vi "NNPC_Eval.vi"(4 "Eval Config":T1={"Extract Good Pixels from Bad"=FALSE, "# bins"=100}, 6 "Dataset(In3D_Out3D)":T28, 8 "error in":errorcluster, 9 "anomaly maps":sgl[][][](array[numeric]), 10 "pred scores":sgl[](array[numeric]), 11 "PCore_Instance in":T2={"Dataset_Stats"={"means"={"R"=0.0, "G"=0.0, "B"=0.0}, "vars"={"R"=0.0, "G"=0.0, "B"=0.0}, "DS_Size"=0}, "NN"={"Name"="", "No of Layers"=0, "mBatch"=0, "Layers"=[], "Dimty"=enum."In1D_Out1D", "Dims_In"={"C"=0, "H"=0, "W"=0}, "Dims_Out"={"C"=0, "H"=0, "W"=0}, "Working_Dir"=path "", "Train?"=FALSE, "Train_Params"={"Optimizer"=enum."SGD", "Beta_1"=0.0, "Beta_2"=0.0, "Weight Decay(L1)"=0.0, "Weight Decay(L2)"=0.0, "Data_Sampling"=enum."Random"}, "LR_Update_Policy"={"Policy_Type"=enum."Manual", "LR0"=0.0, "k"=0.0, "WarmUp_Policy"=enum."Step", "WarmUp_Iter"=0, "WarmUp_Ratio"=0.0}, "Session Data"={"Epochs"=0.0, "Tot_Iter"=0, "LR"=0.0, "LR_iter"=0}, "Ground_truth"={"Y"=variant}, "NNg_hdls"={"cudnn"=0, "cublas"=0, "stream"=0, "curand"=0}, "NN_Device"=enum."CPU", "GPU Id"=0, "Labels"=[], "Receptive Field"=[], "Loss_Type"=enum."None", "Loss_Cfg_Prms"=variant, "NNG_WS"={"NNG_WS_Mem"=refnum, "Max_WS_Size"=0}}, "Device_Config."={"Device"=enum."CPU", "GPU Id"=1}, "PatchCore_Init_CFG"={"BackBone"=enum."WRN_50_2_L2L3", "Out_Layers_Names"=[], "Patch_Size"=0}, "Coreset Params"={"Name"="", "Sampling_Ratio"=0.0, "Startd_idx"=0, "Random_Proj?"=FALSE, "Rnd. Proj. Params"={"Proj._Dim."=0, "Epsilon"=0.9, "Seed"=42}}, "MemBank_Data"={"MemBank"=variant, "MemBank Norm"=variant}} {"NN out"."LR_Update_Policy"."WarmUp_Ratio" min=1; "NN out"."LR_Update_Policy"."WarmUp_Iter" min=1; "NN out"."LR_Update_Policy"."LR0" format="%.7f"; "Dataset_Stats"."vars"."R" format="%#_3g"; "Dataset_Stats"."vars"."G" format="%#_3g"; "Dataset_Stats"."vars"."B" format="%#_3g"; "Dataset_Stats"."means"."R" format="%#_3g"; "Dataset_Stats"."means"."G" format="%#_3g"; "Dataset_Stats"."means"."B" format="%#_3g"}) -> (0 "error out":errorcluster, 1 "Evaluation_Metrics(Pixel)":T30 {"Eval Stats"."Recall(F1_Max)" format="%#_6f"; "Eval Stats"."FPR(F1_Max)" format="%#_6f"; "Eval Stats"."FNR(F1_Max)" format="%#_6f"; "Eval Stats"."Prec.(F1_Max)" format="%#_6f"; "Eval Stats"."F1_Max" format="%#_6f"; "Eval Stats"."AUROC" format="%#_6f"; "Eval Stats"."Scores(Bad)"."Min" format="%#_5g"; "Eval Stats"."Scores(Good)"."Min" format="%#_5g"; "Eval Stats"."Thrshld(F1_Max)" format="%#_6f"}, 2 "Evaluation_Metrics(Image)":T30 {"Eval Stats"."Recall(F1_Max)" format="%#_6f"; "Eval Stats"."FPR(F1_Max)" format="%#_6f"; "Eval Stats"."FNR(F1_Max)" format="%#_6f"; "Eval Stats"."Prec.(F1_Max)" format="%#_6f"; "Eval Stats"."F1_Max" format="%#_6f"; "Eval Stats"."AUROC" format="%#_6f"; "Eval Stats"."Scores(Bad)"."Min" format="%#_5g"; "Eval Stats"."Scores(Good)"."Min" format="%#_5g"; "Eval Stats"."Thrshld(F1_Max)" format="%#_6f"}, 3 "PCore_Instance out":T2={"Dataset_Stats"={"means"={"R"=0.0, "G"=0.0, "B"=0.0}, "vars"={"R"=0.0, "G"=0.0, "B"=0.0}, "DS_Size"=0}, "NN"={"Name"="", "No of Layers"=0, "mBatch"=0, "Layers"=[], "Dimty"=enum."In1D_Out1D", "Dims_In"={"C"=0, "H"=0, "W"=0}, "Dims_Out"={"C"=0, "H"=0, "W"=0}, "Working_Dir"=path "", "Train?"=FALSE, "Train_Params"={"Optimizer"=enum."SGD", "Beta_1"=0.0, "Beta_2"=0.0, "Weight Decay(L1)"=0.0, "Weight Decay(L2)"=0.0, "Data_Sampling"=enum."Random"}, "LR_Update_Policy"={"Policy_Type"=enum."Manual", "LR0"=0.0, "k"=0.0, "WarmUp_Policy"=enum."Step", "WarmUp_Iter"=0, "WarmUp_Ratio"=0.0}, "Session Data"={"Epochs"=0.0, "Tot_Iter"=0, "LR"=0.0, "LR_iter"=0}, "Ground_truth"={"Y"=variant}, "NNg_hdls"={"cudnn"=0, "cublas"=0, "stream"=0, "curand"=0}, "NN_Device"=enum."CPU", "GPU Id"=0, "Labels"=[], "Receptive Field"=[], "Loss_Type"=enum."None", "Loss_Cfg_Prms"=variant, "NNG_WS"={"NNG_WS_Mem"=refnum, "Max_WS_Size"=0}}, "Device_Config."={"Device"=enum."CPU", "GPU Id"=1}, "PatchCore_Init_CFG"={"BackBone"=enum."WRN_50_2_L2L3", "Out_Layers_Names"=[], "Patch_Size"=0}, "Coreset Params"={"Name"="", "Sampling_Ratio"=0.0, "Startd_idx"=0, "Random_Proj?"=FALSE, "Rnd. Proj. Params"={"Proj._Dim."=0, "Epsilon"=0.9, "Seed"=42}}, "MemBank_Data"={"MemBank"=variant, "MemBank Norm"=variant}} {"NN out"."LR_Update_Policy"."WarmUp_Ratio" min=1; "NN out"."LR_Update_Policy"."WarmUp_Iter" min=1; "NN out"."LR_Update_Policy"."LR0" format="%.7f"; "Dataset_Stats"."vars"."R" format="%#_3g"; "Dataset_Stats"."vars"."G" format="%#_3g"; "Dataset_Stats"."vars"."B" format="%#_3g"; "Dataset_Stats"."means"."R" format="%#_3g"; "Dataset_Stats"."means"."G" format="%#_3g"; "Dataset_Stats"."means"."B" format="%#_3g"}, 5 "dT_Eval":dbl=0.3182995500001198 format="%#_4ps")   [LabVIEW 2020, in "PatchCore_AddOn.lvlib"]
uses:
  PatchCore_AddOn.lvlib
  Controls/Evaluation_Metrics.ctl
  Controls/Eval_Results.ctl
  Controls/MinMax.ctl
  <vilib>/Ngene/Deep Learning Toolkit/Toolkit/NN_Data/API/DataSet/DataSet_Types/NN_DataSet(In3D_Out3D).ctl
  <vilib>/Ngene/Deep Learning Toolkit/Toolkit/NN_Data/API/NN_Dims(C,H,W).ctl
  <vilib>/Ngene/Deep Learning Toolkit/Toolkit/NN_Data/Controls/DataRef_Types/4D/NN_Data_ref(4D_SGL).ctl
  Controls/NNPC_Instance.ctl
  Controls/NNPC_DS_Stats.ctl
  Controls/Image_Stats_RGB.ctl
  <vilib>/Ngene/Deep Learning Toolkit/Toolkit/NN_Network/Controls/NN.ctl
  <vilib>/Ngene/Deep Learning Toolkit/Toolkit/NN_Layers/Controls/NN_Layer_ref.ctl
  <vilib>/Ngene/Deep Learning Toolkit/Toolkit/NN_Layers/Controls/NN_Layer.ctl
  <vilib>/Ngene/Deep Learning Toolkit/Toolkit/NN_Layers/Controls/NN_Layer_Type.ctl
  <vilib>/Ngene/Deep Learning Toolkit/Toolkit/NN_Layers/Controls/NN_Layer_Metrics.ctl
  <vilib>/Ngene/Deep Learning Toolkit/Toolkit/NN_Network/Controls/NN_Device.ctl
  <vilib>/Ngene/Deep Learning Toolkit/Toolkit/NNg/cuda/Controls/nng_cuda_handles.ctl
  <vilib>/Ngene/Deep Learning Toolkit/Toolkit/NN_Layers/Controls/NN_Layer_Dimty.ctl
  <vilib>/Ngene/Deep Learning Toolkit/Toolkit/NN_Layers/Controls/NN_Layer_RF_State.ctl
  <vilib>/Ngene/Deep Learning Toolkit/Toolkit/NN_Data/API/NN_Dims(V,H).ctl
  <vilib>/Ngene/Deep Learning Toolkit/Toolkit/NN_Network/Controls/NN_In_Out_Dim-ty.ctl
  <vilib>/Ngene/Deep Learning Toolkit/Toolkit/NN_Train/Controls/NN_Train_Params.ctl
  <vilib>/Ngene/Deep Learning Toolkit/Toolkit/NN_Train/Controls/NN_Train_Optimizer.ctl
  <vilib>/Ngene/Deep Learning Toolkit/Toolkit/NN_Train/Controls/NN_Train_Data_Sampling.ctl
  <vilib>/Ngene/Deep Learning Toolkit/Toolkit/NN_Train/Controls/NN_LR_Policy_Cfg.ctl
  <vilib>/Ngene/Deep Learning Toolkit/Toolkit/NN_Train/Controls/NN_LR_Policy_Type.ctl
  <vilib>/Ngene/Deep Learning Toolkit/Toolkit/NN_Train/Controls/NN_Train_Session_Data.ctl
  <vilib>/Ngene/Deep Learning Toolkit/Toolkit/NN_Data/Controls/NN_Ground_truth.ctl
  <vilib>/Ngene/Deep Learning Toolkit/Toolkit/NN_Train/Controls/NN_Loss_Type.ctl
  <vilib>/Ngene/Deep Learning Toolkit/Toolkit/NNg/Network/WS/Controls/NNG_WS.ctl
  <vilib>/Ngene/Deep Learning Toolkit/Toolkit/NNg/Network/WS/Controls/NNg_WS_Mem_DVR.ctl
  <vilib>/Ngene/Deep Learning Toolkit/Toolkit/NNg/cuda/Controls/cuda_Mem_desc.ctl
  Controls/NNPC_Device.ctl
  Controls/NNPC_Init_CFG.ctl
  Controls/NNPC_BackBone_Selector.ctl
  Controls/NNPC_Coreset_Params.ctl
  Controls/NNPC_Random_Projection_CFG.ctl
  Controls/MemBank_and_Norm_Variants.ctl
  Controls/Eval_Config.ctl
  <vilib>/Ngene/Deep Learning Toolkit/Toolkit/Deep_Learning_Toolkit_by_Ngene.lvlib
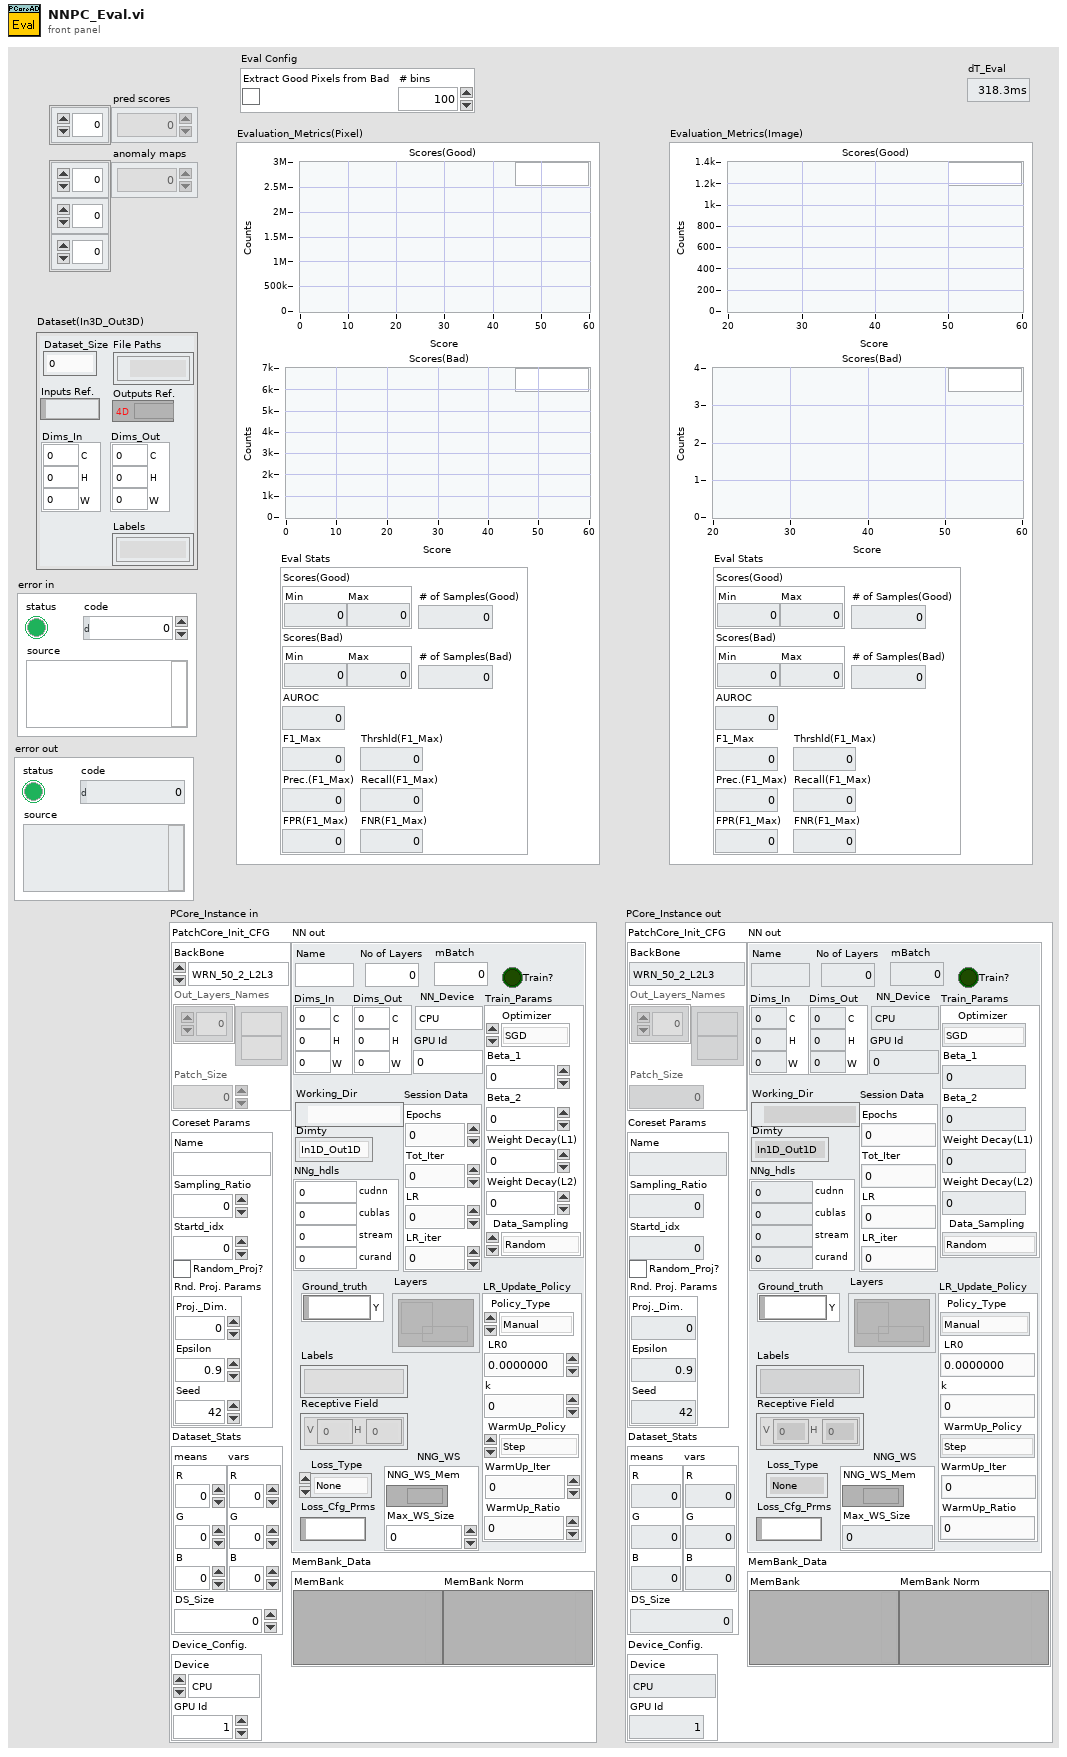
[diagram p1: front panel]
types:
  T1 = typedef "PatchCore_AddOn.lvlib/Eval_Config.ctl" = cluster{"Extract Good Pixels from Bad":bool, "# bins":i32}
  T2 = typedef "PatchCore_AddOn.lvlib/NNPC_Instance.ctl" = cluster{"Dataset_Stats":T3, "NN":T5, "Device_Config.":T22, "PatchCore_Init_CFG":T23, "Coreset Params":T25, "MemBank_Data":T27}
  T3 = typedef "PatchCore_AddOn.lvlib/NNPC_DS_Stats.ctl" = cluster{"means":T4, "vars":T4, "DS_Size":i32}
  T4 = typedef "PatchCore_AddOn.lvlib/Image_Stats_RGB.ctl" = cluster{"R":sgl, "G":sgl, "B":sgl}
  T5 = typedef "Deep_Learning_Toolkit_by_Ngene.lvlib/NN.ctl" = cluster{"Name":string, "No of Layers":i32, "mBatch":i32, "Layers":T6[], "Dimty":T7, "Dims_In":T8, "Dims_Out":T8, "Working_Dir":path, "Train?":bool, "Train_Params":T9, "LR_Update_Policy":T12, "Session Data":T14, "Ground_truth":T15, "NNg_hdls":T16, "NN_Device":T17, "GPU Id":i32, "Labels":string[], "Receptive Field":T18[], "Loss_Type":T19, "Loss_Cfg_Prms":variant, "NNG_WS":T20}
  T6 = typedef "Deep_Learning_Toolkit_by_Ngene.lvlib/NN_Layer_ref.ctl" = refnum<data-value>
  T7 = typedef "Deep_Learning_Toolkit_by_Ngene.lvlib/NN_In_Out_Dim-ty.ctl" = enum8{"In1D_Out1D", "In3D_Out1D", "In3D_Out3D", "In3D_OutBBox"}
  T8 = typedef "Deep_Learning_Toolkit_by_Ngene.lvlib/NN_Dims(C,H,W).ctl" = cluster{"C":i32, "H":i32, "W":i32}
  T9 = typedef "Deep_Learning_Toolkit_by_Ngene.lvlib/NN_Train_Params.ctl" = cluster{"Optimizer":T10, "Beta_1":sgl, "Beta_2":sgl, "Weight Decay(L1)":sgl, "Weight Decay(L2)":sgl, "Data_Sampling":T11}
  T10 = typedef "Deep_Learning_Toolkit_by_Ngene.lvlib/NN_Train_Optimizer.ctl" = enum16{"SGD", "Adam", "Adagrad", "Adadelta", "RMSProp", "Nesterov"}
  T11 = typedef "Deep_Learning_Toolkit_by_Ngene.lvlib/NN_Train_Data_Sampling.ctl" = enum16{"Random", "Sequential"}
  T12 = typedef "Deep_Learning_Toolkit_by_Ngene.lvlib/NN_LR_Policy_Cfg.ctl" = cluster{"Policy_Type":T13, "LR0":dbl, "k":sgl, "WarmUp_Policy":enum16{"Step", "Ramp"}, "WarmUp_Iter":i32, "WarmUp_Ratio":sgl}
  T13 = typedef "Deep_Learning_Toolkit_by_Ngene.lvlib/NN_LR_Policy_Type.ctl" = enum16{"Manual", "Step", "Exp", "1/t"}
  T14 = typedef "Deep_Learning_Toolkit_by_Ngene.lvlib/NN_Train_Session_Data.ctl" = cluster{"Epochs":sgl, "Tot_Iter":i32, "LR":sgl, "LR_iter":i32}
  T15 = typedef "Deep_Learning_Toolkit_by_Ngene.lvlib/NN_Ground_truth.ctl" = cluster{"Y":variant}
  T16 = typedef "Deep_Learning_Toolkit_by_Ngene.lvlib/nng_cuda_handles.ctl" = cluster{"cudnn":u64, "cublas":u64, "stream":u64, "curand":u64}
  T17 = typedef "Deep_Learning_Toolkit_by_Ngene.lvlib/NN_Device.ctl" = enum16{"CPU", "GPU"}
  T18 = typedef "Deep_Learning_Toolkit_by_Ngene.lvlib/NN_Dims(V,H).ctl" = cluster{"V":i32, "H":i32}
  T19 = typedef "Deep_Learning_Toolkit_by_Ngene.lvlib/NN_Loss_Type.ctl" = enum16{"None", "MSE", "CrossEntropy", "YOLO_v2", "YOLO_v4"}
  T20 = typedef "Deep_Learning_Toolkit_by_Ngene.lvlib/NNG_WS.ctl" = cluster{"NNG_WS_Mem":T21, "Max_WS_Size":i64}
  T21 = typedef "Deep_Learning_Toolkit_by_Ngene.lvlib/NNg_WS_Mem_DVR.ctl" = refnum<data-value>
  T22 = typedef "PatchCore_AddOn.lvlib/NNPC_Device.ctl" = cluster{"Device":T17, "GPU Id":i32}
  T23 = typedef "PatchCore_AddOn.lvlib/NNPC_Init_CFG.ctl" = cluster{"BackBone":T24, "Out_Layers_Names":string[], "Patch_Size":u32}
  T24 = typedef "PatchCore_AddOn.lvlib/NNPC_BackBone_Selector.ctl" = enum16{"WRN_50_2_L2L3"}
  T25 = typedef "PatchCore_AddOn.lvlib/NNPC_Coreset_Params.ctl" = cluster{"Name":string, "Sampling_Ratio":sgl, "Startd_idx":i32, "Random_Proj?":bool, "Rnd. Proj. Params":T26}
  T26 = typedef "PatchCore_AddOn.lvlib/NNPC_Random_Projection_CFG.ctl" = cluster{"Proj._Dim.":i32, "Epsilon":sgl, "Seed":i32}
  T27 = typedef "PatchCore_AddOn.lvlib/MemBank_and_Norm_Variants.ctl" = cluster{"MemBank":variant, "MemBank Norm":variant}
  T28 = typedef "Deep_Learning_Toolkit_by_Ngene.lvlib/NN_DataSet(In3D_Out3D).ctl" = cluster{"Dataset_Size":i32, "Dims_In":T8, "Labels":string[], "File Paths":path[], "Outputs Ref.":T29, "Inputs Ref.":variant, "Dims_Out":T8}
  T29 = typedef "Deep_Learning_Toolkit_by_Ngene.lvlib/NN_Data_ref(4D_SGL).ctl" = refnum<data-value>
  T30 = typedef "PatchCore_AddOn.lvlib/Evaluation_Metrics.ctl" = cluster{"Scores(Good)":cluster{"X Values":dbl[], "Histogram: h(x)":i32[]}, "Scores(Bad)":cluster{"X Values":dbl[], "Histogram: h(x)":i32[]}, "Eval Stats":T31}
  T31 = typedef "PatchCore_AddOn.lvlib/Eval_Results.ctl" = cluster{"Scores(Good)":T32, "Scores(Bad)":T32, "# of Samples(Good)":i32, "# of Samples(Bad)":i32, "AUROC":sgl, "F1_Max":sgl, "Thrshld(F1_Max)":sgl, "Prec.(F1_Max)":sgl, "Recall(F1_Max)":sgl, "FPR(F1_Max)":sgl, "FNR(F1_Max)":sgl}
  T32 = typedef "PatchCore_AddOn.lvlib/MinMax.ctl" = cluster{"Min":sgl, "Max":sgl}
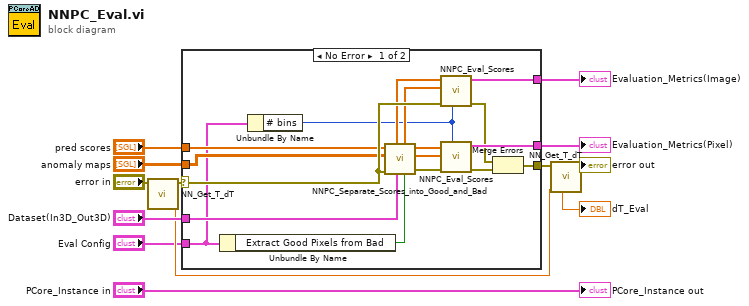
[diagram p0: block diagram]
diagram:
  n1 = call <vilib>:"NN_Get_T_dT.vi"("error in (no error)"="error in") -> ("T_out"=w6:dbl, "error out"=w8:errorcluster)  [unwired: 6 in, 1 out]
  n2 = case shown="No Error" w8 {
    selector: w8 -> [w25 w31]
    tunnel: [w30 _] -> w13
    tunnel: [w29 _] -> w12
    tunnel: "Dataset(In3D_Out3D)" -> [w28 _]
    tunnel: [w21 w31] -> w9
    tunnel: "Eval Config" -> [w15 _]
    tunnel: "pred scores" -> [w18 _]
    tunnel: "anomaly maps" -> [w17 _]
    frame No Error {
      n3 = Unbundle By Name(w15) -> ("Extract Good Pixels from Bad"=w16:bool)
      n4 = Unbundle By Name(w15) -> ("# bins"=w14:i32)
      n5 = call "NNPC_Separate_Scores_into_Good_and_Bad.vi"("Extract Good Pixels from Bad Images"=w16, "Dataset"=w28, "error in"=w25, "Pixel Scores"=w17, "Image Scores"=w18) -> ("error out"=w24:errorcluster, "Bad Pixel Scores"=w27:sgl[], "Good Pixel Scores"=w26:sgl[], "Bad Image Scores"=w19:sgl[], "Good Image Scores"=w20:sgl[])  [unwired: 2 in]
      n6 = call "NNPC_Eval_Scores.vi"("# bins"=w14, "error in(no errror)"=w25, "Scores(Bad)"=w19, "Scores(Good)"=w20) -> ("error out"=w23:errorcluster, "Evaluation_Metrics"=w29:T30)  [unwired: 5 in, 1 out]
      n7 = call "NNPC_Eval_Scores.vi"("# bins"=w14, "error in(no errror)"=w24, "Scores(Bad)"=w27, "Scores(Good)"=w26) -> ("error out"=w22:errorcluster, "Evaluation_Metrics"=w30:T30)  [unwired: 5 in, 1 out]
      n8 = Merge Errors(w23, w22) -> (w21:errorcluster)
    }
    frame Error {
    }
  }
  "Evaluation_Metrics(Image)" <- w12
  "Evaluation_Metrics(Pixel)" <- w13
  n9 = call <vilib>:"NN_Get_T_dT.vi"("T_in"=w6, "error in (no error)"=w9) -> ("error out"=→"error out":errorcluster, "dT"=→"dT_Eval":dbl)  [unwired: 5 in, 1 out]
  "PCore_Instance out" <- "PCore_Instance in"
